vi "Set oscillating rate.vi"(4 "Switch enhance factor":dbl=0.5 format="%#.4f", 6 "Pump 1 reaction oscillate rate (ml/min)":dbl=0.5 format="%#.4f", 10 "Direaction":enum16{"Forward", "Backward"}(ring), 11 "Pump COM":refnum<visa-resource-name>) -> (0 "error out":errorcluster, 3 "VISA resource name out":refnum<visa-resource-name>)   [LabVIEW 2017]
uses:
  <instrlib>/Harvard Apparatus PHD Ultra Series/Harvard Apparatus PHD Ultra Series.lvlib
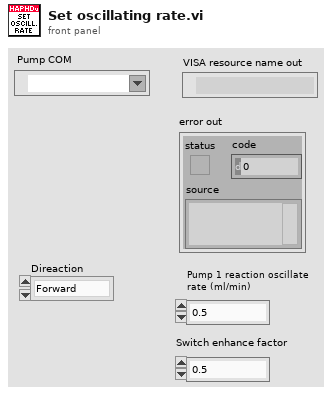
[diagram p1: front panel]
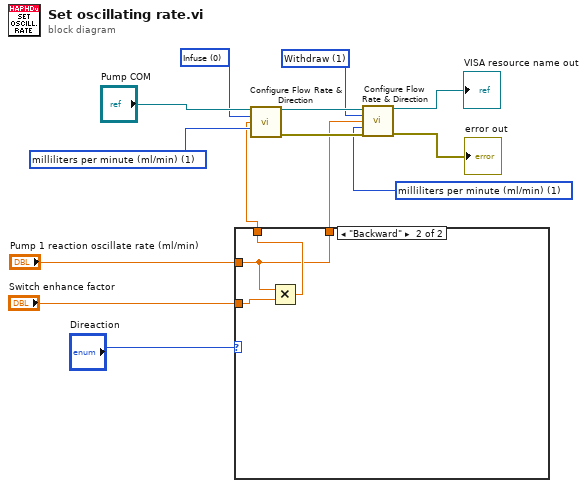
[diagram p0: block diagram]
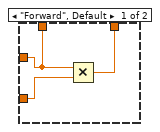
[diagram p2: hidden frame]
diagram:
  w6 = u32 1 items=["milliliters per hour (ml/hr)", "milliliters per minute (ml/min)", "milliliters per second (ml/sec)", "microliters per hour (ul/hr)", "microliters per minute (ul/min)", "microliters per second (ul/sec)", "nanoliters per hour (nl/hr)", "nanoliters per minute (nl/min)", "nanoliters per second (nl/sec)", "picoliters per hour (pl/hr)", "picoliters per minute (pl/min)", "picoliters per second (pl/sec)"] ("Flow Rate Units (1:ml/min)")
  w7 = u32 1 items=["milliliters per hour (ml/hr)", "milliliters per minute (ml/min)", "milliliters per second (ml/sec)", "microliters per hour (ul/hr)", "microliters per minute (ul/min)", "microliters per second (ul/sec)", "nanoliters per hour (nl/hr)", "nanoliters per minute (nl/min)", "nanoliters per second (nl/sec)", "picoliters per hour (pl/hr)", "picoliters per minute (pl/min)", "picoliters per second (pl/sec)"] ("Flow Rate Units (1:ml/min)")
  w10 = u16 1 items=["Infuse", "Withdraw"] ("Pump Direction (0:Infuse)")
  w11 = u16 0 items=["Infuse", "Withdraw"] ("Pump Direction (0:Infuse)")
  n1 = case shown="\"Backward\"" "Direaction" {
    tunnel: "Pump 1 reaction oscillate rate (ml/min)" -> [w15 w19]
    tunnel: "Switch enhance factor" -> [w16 w18]
    tunnel: [w17 w19] -> w2
    tunnel: [w15 w20] -> w1
    frame "Forward", Default {
      n2 = Multiply(x=w15, y=w16) -> (x*y=w17:dbl)
    }
    frame "Backward" {
      n3 = Multiply(x=w19, y=w18) -> (x*y=w20:dbl)
    }
  }
  n4 = call <instrlib>:"Configure Flow Rate & Direction.vi"("VISA resource name"="Pump COM", "Pump Direction (0:Infuse)"=w11, "Flow Rate (5.00)"=w1, "Flow Rate Units (1:ml/min)"=w7) -> ("VISA resource name out"=w13:refnum<visa-resource-name>, "error out"=w14:errorcluster)  [unwired: 10 in]
  n5 = call <instrlib>:"Configure Flow Rate & Direction.vi"("VISA resource name"=w13, "Pump Direction (0:Infuse)"=w10, "Flow Rate (5.00)"=w2, "Flow Rate Units (1:ml/min)"=w6, "error in (no error)"=w14) -> ("VISA resource name out"=→"VISA resource name out":refnum<visa-resource-name>, "error out"=→"error out":errorcluster)  [unwired: 9 in]
